vi "CreateFolder.vi"(0 "object in":refnum<class "Experiment.lvclass">, 5 "error in (no error)":errorcluster) -> (14 "object out":refnum<class "Experiment.lvclass">, 16 "FolderPath":path, 19 "error out":errorcluster)   [LabVIEW 2019, in "Experiment.lvclass"]
uses:
  Experiment.lvclass
  Experiment.lvclass/Experiment.ctl
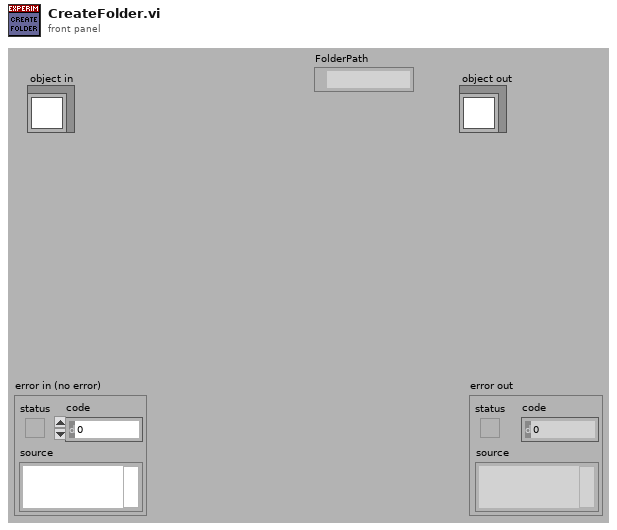
[diagram p1: front panel]
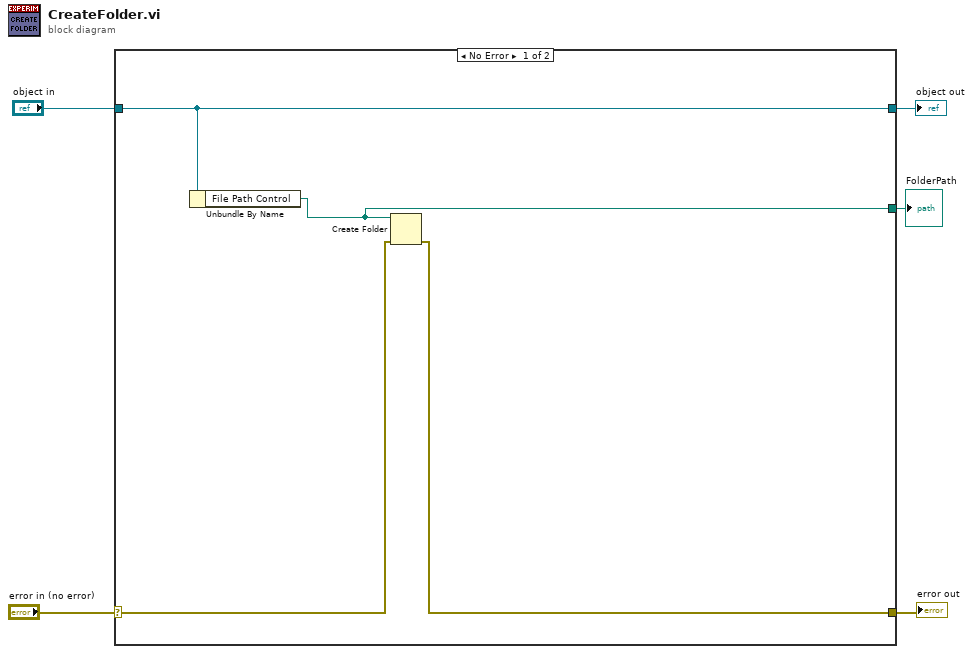
[diagram p0: block diagram]
diagram:
  n1 = case shown="No Error" "error in (no error)" {
    selector: "error in (no error)" -> [w8 w11]
    tunnel: [w7 w11] -> w4
    tunnel: [w9 w10] -> w2
    tunnel: "object in" -> [w9 w10]
    tunnel: [w6 _] -> w1
    frame No Error {
      n2 = Unbundle By Name(w9) -> ("File Path Control"=w6:path)
      n3 = Create Folder(path (use dialog)=w6, error in=w8) -> (error out=w7:errorcluster)  [unwired: 1 in, 2 out]
    }
    frame Error {
    }
  }
  "error out" <- w4
  "object out" <- w2
  "FolderPath" <- w1
